vi "Get Physical Units__ogtk.vi"(8 "error in (no error)":errorcluster, 10 "Float or Array of Floats":variant) -> (0 "error out":errorcluster, 2 "Physical Units":T1[](array[typedef]))   [LabVIEW 2016]
doc: "Returns the physical units of the variant input (number or array)."
uses:
  <userlib>/_OpenG.lib/lvdata/lvdata.llb/Physical Units__ogtk.ctl
panel:
  # "[OpenG VI Tags] ***Do Not Remove***"
  # "Please visit http://www.OpenG.org to learn about the\nOpen Source LabVIEW software movement.\n\nNOTICE -- YOU MUST LEAVE THIS NOTICE IN PLACE.  PER THE TERMS OF THE LICENSE BELOW, YOU MAY SUBLICENSE THIS SOFTWARE \nIN ANY WAY THAT DOES NOT CONFLICT WITH THIS LICENSE.\n\n### BSD License (http://www.opensource.org/licenses/bsd-license.php) Begin ###\n \nCopyright (c) 2002, Jean-Pierre Drolet <drolet_jp@hotmail.com>\nCopyright (c) 2002-2006, Jim Kring <jim@jimkring.com>\n\nAll rights reserved.\n\nRedistribution and use in source and binary forms, with or without modification, are permitted provided that the following conditions are met:\n\n    * Redistributions of source code must retain the above copyright notice, this list of conditions and the following disclaimer.\n    * Redistributions in binary form must reproduce the above copyright notice, this list of conditions and the following disclaimer in the \n       documentation and/or other materials provided with the distribution.\n    * Neither the name of SciWare, James Kring, Inc., nor the names of its contributors may be used to endorse or promote products derived \n       from this software without specific prior written permission.\n\nTHIS SOFTWARE IS PROVIDED BY THE COPYRIGHT HOLDERS AND CONTRIBUTORS \"AS IS\" AND ANY EXPRESS OR IMPLIED WARRANTIES, \nINCLUDING, BUT NOT LIMITED TO, THE IMPLIED WARRANTIES OF MERCHANTABILITY AND FITNESS FOR A PARTICULAR PURPOSE ARE \nDISCLAIMED. IN NO EVENT SHALL THE COPYRIGHT OWNER OR CONTRIBUTORS BE LIABLE FOR ANY DIRECT, INDIRECT, INCIDENTAL,\n SPECIAL, EXEMPLARY, OR CONSEQUENTIAL DAMAGES (INCLUDING, BUT NOT LIMITED TO, PROCUREMENT OF SUBSTITUTE GOODS OR \nSERVICES; LOSS OF USE, DATA, OR PROFITS; OR BUSINESS INTERRUPTION) HOWEVER CAUSED AND ON ANY THEORY OF LIABILITY, \nWHETHER IN CONTRACT, STRICT LIABILITY, OR TORT (INCLUDING NEGLIGENCE OR OTHERWISE) ARISING IN ANY WAY OUT OF THE USE \nOF THIS SOFTWARE, EVEN IF ADVISED OF THE POSSIBILITY OF SUCH DAMAGE.\n\n### BSD License End ###"
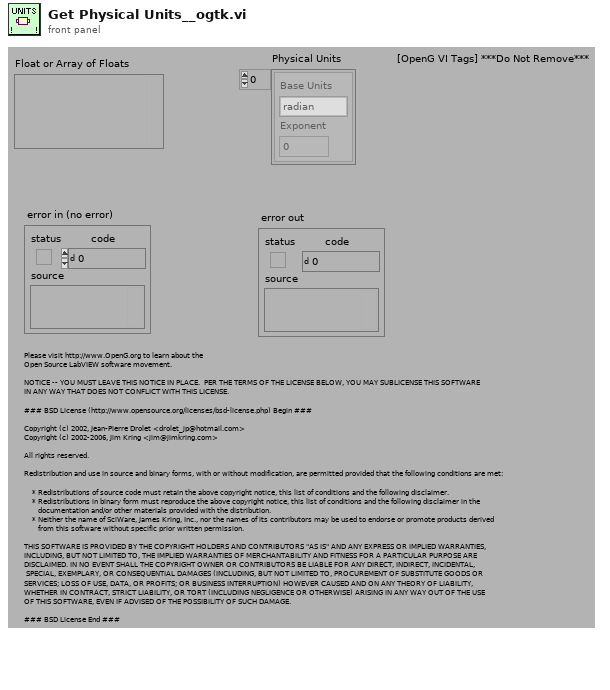
[diagram p1: front panel]
types:
  T1 = typedef "Physical Units__ogtk.ctl" = cluster{"Base Units":enum16{"radian", "steradian", "second", "meter", "kilogram", "ampere", "kelvin", "mole", "candela"}, "Exponent":i16}
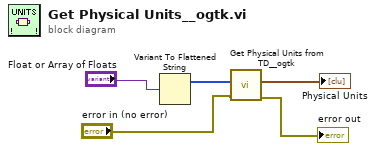
[diagram p0: block diagram]
diagram:
  n1 = Variant To Flattened String(Variant="Float or Array of Floats") -> (1:w1:i16[])  [unwired: 1 out]
  n2 = call <userlib>:"Get Physical Units from TD__ogtk.vi"("error in (no error)"="error in (no error)", "Float or Array Type Descriptor"=w1) -> ("error out"=→"error out":errorcluster, "Physical Units"=→"Physical Units":T1[])  [unwired: 8 in]
